vi "MokoInfo_Registration.vi"(8 "Error In":errorcluster, 11 "Registration in":T1) -> (0 "Error Out":errorcluster, 3 "Registration out":T1)   [LabVIEW 2018]
uses:
  MokoInfo_Registration.ctl
panel:
  in  "Contact Person":string caption="String"
  in  "Email":string caption="String"
  in  "Phone number":string caption="String"
  in  "INN":string caption="String"
  in  "OGRN":string caption="String"
  in  "Addres":string caption="String"
  in  "Customer":string caption="String"
  in  "Save":bool
  # "Registration of the customer:"
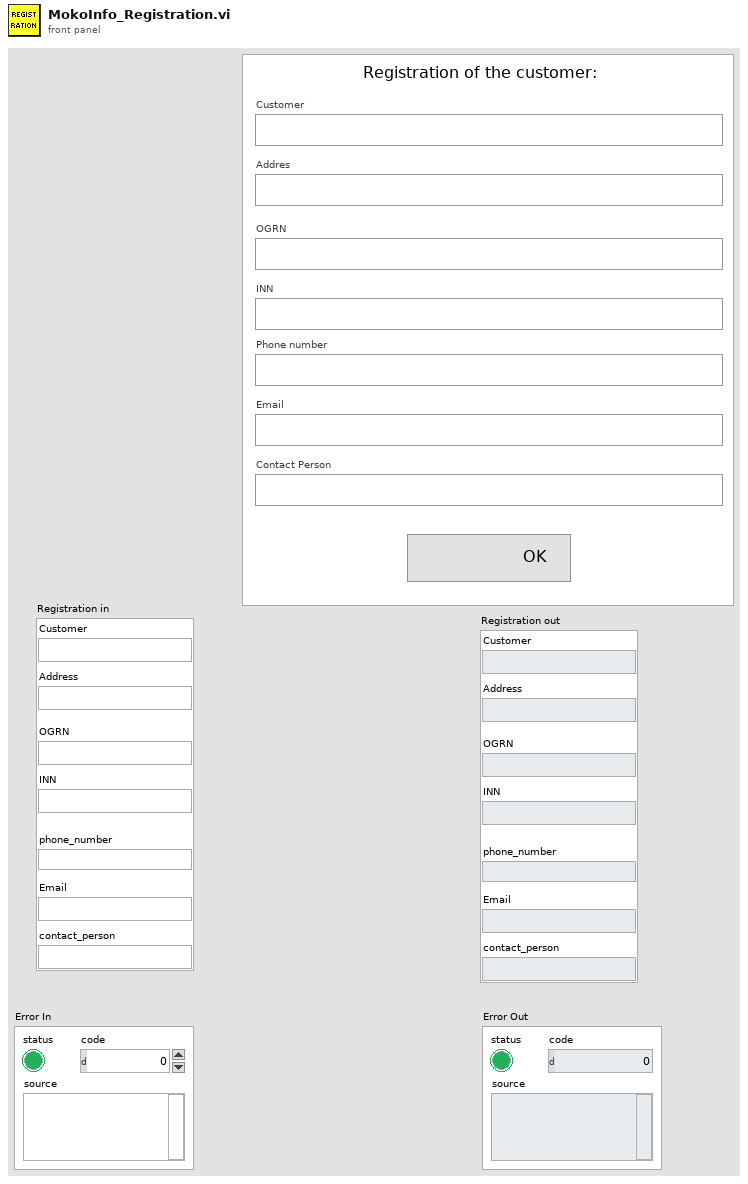
[diagram p1: front panel]
types:
  T1 = typedef "MokoInfo_Registration.ctl" = cluster{"name_of_the_customer":string, "the_address_of_the_customer":string, "OGRN":string, "INN":string, "phone_number":string, "Email":string, "contact_person":string}
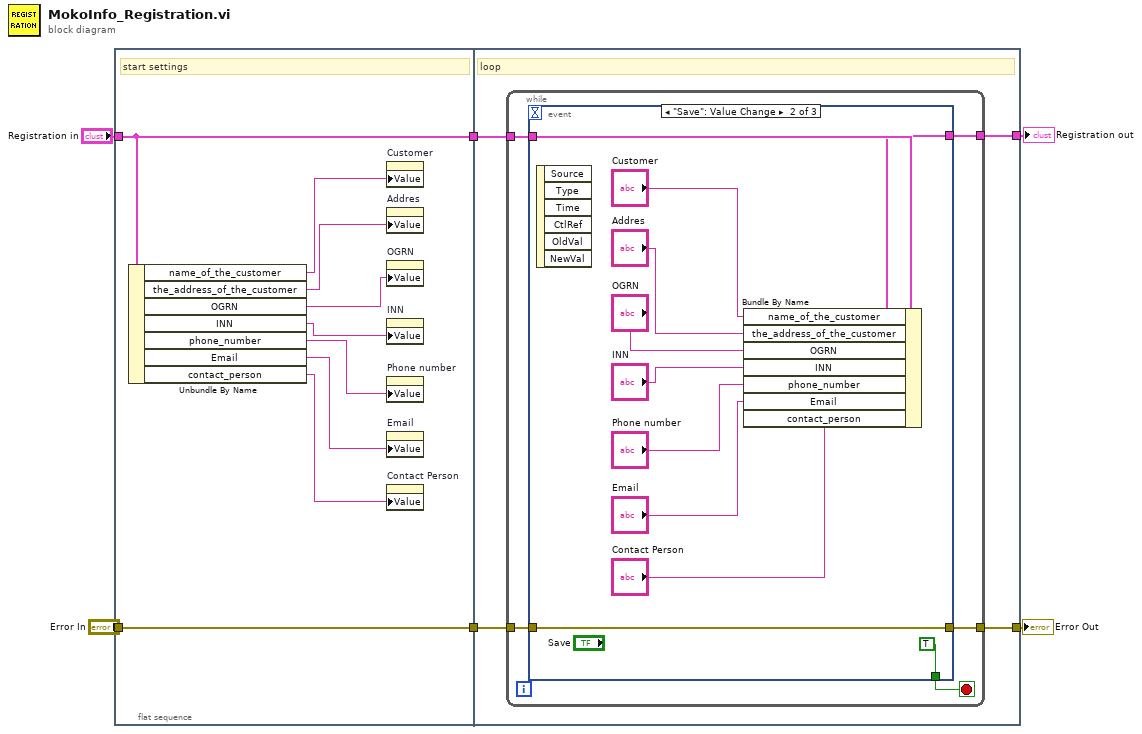
[diagram p0: block diagram]
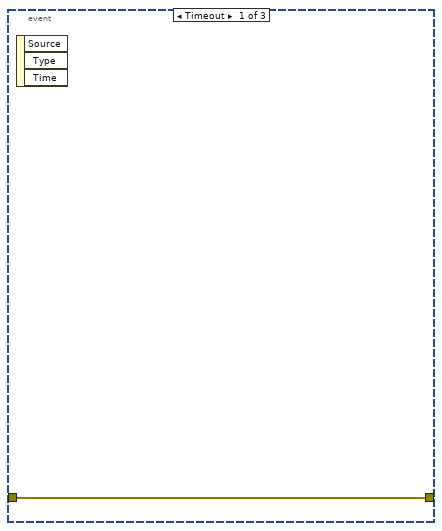
[diagram p2: hidden frame]
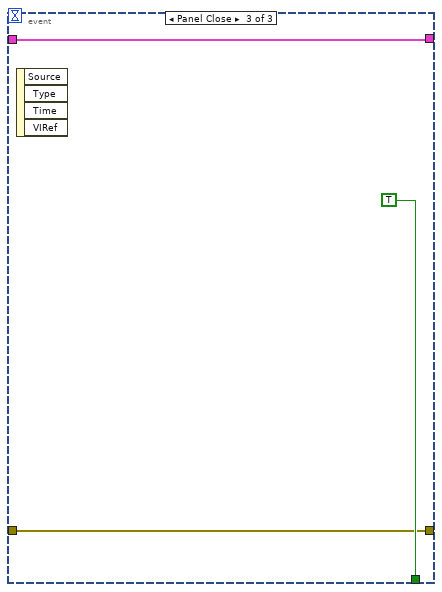
[diagram p3: hidden frame]
diagram:
  n1 = flat-sequence {
    tunnel: [w15] -> w6
    tunnel: "Registration in" -> [w15]
    tunnel: [w14] -> w3
    tunnel: "Error In" -> [w14]
    tunnel: w6 -> [w19]
    tunnel: [w18] -> w4
    tunnel: w3 -> [w16]
    tunnel: [w17] -> w1
    frame #0 {
      # "start settings"
      n2 = Unbundle By Name(w15) -> ("name_of_the_customer"=w13:string, "the_address_of_the_customer"=w12:string, "OGRN"=w11:string, "INN"=w10:string, "phone_number"=w9:string, "Email"=w8:string, "contact_person"=w7:string)
      n3 = property on="Customer" class="Str"("Value"=w13) -> ()  [unwired: 2 in, 2 out]
      n4 = property on="Addres" class="Str"("Value"=w12) -> ()  [unwired: 2 in, 2 out]
      n5 = property on="OGRN" class="Str"("Value"=w11) -> ()  [unwired: 2 in, 2 out]
      n6 = property on="INN" class="Str"("Value"=w10) -> ()  [unwired: 2 in, 2 out]
      n7 = property on="Phone number" class="Str"("Value"=w9) -> ()  [unwired: 2 in, 2 out]
      n8 = property on="Email" class="Str"("Value"=w8) -> ()  [unwired: 2 in, 2 out]
      n9 = property on="Contact Person" class="Str"("Value"=w7) -> ()  [unwired: 2 in, 2 out]
    }
    frame #1 {
      # "loop"
      n10 = while {
        tunnel: w19 -> [w23]
        tunnel: [w22] -> w18
        tunnel: [w21] -> w17
        tunnel: w16 -> [w20]
        stop <- w24 stop-if-true
        n11 = event shown="[1] \"Save\": Value Change" {
          selector: _ -> [_ _ _]
          dyn-events: _ -> [_ _ _]
          timeout: _ -> [_ _ _]
          tunnel: [_ TRUE TRUE] -> w24
          tunnel: w23 -> [_ w35 w38]
          tunnel: [_ w34 w38] -> w22
          tunnel: [w25 w33 w37] -> w21
          tunnel: w20 -> [w25 w33 w37]
          event Timeout {
            n12 = event-data() -> ()  [unwired: 1 in, 3 out]
          }
          event "Save": Value Change {
            n13 = event-data() -> ()  [unwired: 1 in, 6 out]
            n14 = Bundle By Name(cluster=w35, "name_of_the_customer"="Customer", "the_address_of_the_customer"="Addres", "OGRN"="OGRN", "INN"="INN", "phone_number"="Phone number", "Email"="Email", "contact_person"="Contact Person") -> (w34:T1)
          }
          event Panel Close {
            n15 = event-data() -> ()  [unwired: 1 in, 4 out]
          }
        }
      }
    }
  }
  "Registration out" <- w4
  "Error Out" <- w1
